vi "CalcSampleRVSplitterBox.vi"(8 "Rp":dbl format="%#_13g", 9 "Rl":dbl format="%#_13g", 10 "Source Voltage (V)":dbl format="%#_13g", 11 "Sample Current (A)":dbl format="%#_13g") -> (0 "Sample Resistance (Ohms)":dbl, 3 "Sample Voltage (V)":dbl)   [LabVIEW 2016]
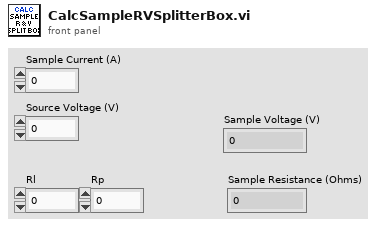
[diagram p1: front panel]
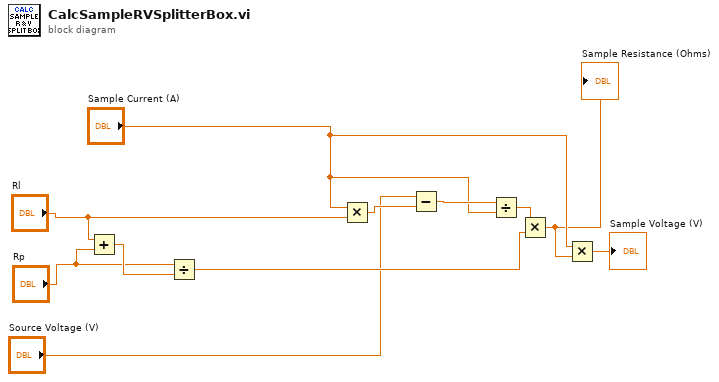
[diagram p0: block diagram]
diagram:
  n1 = Add(x="Rl", y="Rp") -> (x+y=w9:dbl)
  n2 = Divide(x="Rp", y=w9) -> (x/y=w6:dbl)
  n3 = Multiply(x="Sample Current (A)", y="Rl") -> (x*y=w11:dbl)
  n4 = Subtract(x="Source Voltage (V)", y=w11) -> (x-y=w10:dbl)
  n5 = Divide(x=w10, y="Sample Current (A)") -> (x/y=w7:dbl)
  n6 = Multiply(x=w7, y=w6) -> (x*y=w2:dbl)
  "Sample Resistance (Ohms)" <- w2
  n7 = Multiply(x="Sample Current (A)", y=w2) -> (x*y=→"Sample Voltage (V)":dbl)
